vi "QueryServer_Query_GetRequest.vi"(0 "gRPCid":T1, 3 "error in (no error)":errorcluster) -> (7 "gRPCid out":T1, 8 "query":string, 10 "error out":errorcluster)   [LabVIEW 2019]
uses:
  QueryServer_gRPCid.ctl
  QueryServer_QueryRequest.ctl
  Debug/labview_query_server.dll
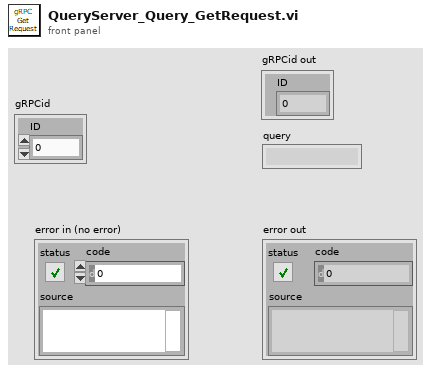
[diagram p1: front panel]
types:
  T1 = typedef "QueryServer_gRPCid.ctl" = cluster{"ID":u64}
  T2 = typedef "QueryServer_QueryRequest.ctl" = cluster{"query":string}
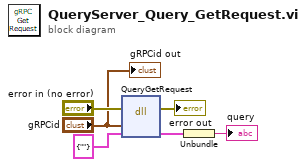
[diagram p0: block diagram]
diagram:
  n1 = dll-call lib="C:/dev/labview-grpc-query-server/Debug/labview_query_server.dll" fn="QueryGetRequest"(error in="error in (no error)", "id"="gRPCid", "data"=T2 {"query"=""} ("QueryRequest")) -> (error out=→"error out":errorcluster, "data"=w2:T2)  [unwired: 4 in, 1 out]
  n2 = Unbundle(w2) -> ("query"=→"query":string)
  "gRPCid out" <- "gRPCid"
